vi "DestroyRequestEvents.vi"(8 "error in (no error)":errorcluster) -> (0 "error out":errorcluster)   [LabVIEW 2018, in "MyPlugins.lvlib"]
doc: "Closes the user events generated that describe which requests can be sent to the module."
uses:
  MyPlugins.lvlib
  PluginsShared/clRequestEvents.ctl
  PluginsShared/clEventType.ctl
  PluginsShared/PluginsShared.lvlib
panel:
  out "clRequestEvents":T1
  # "If you want to add other Request Events, open this typedef, copy an existing event and rename it to your Request name.\n\nNext create a typedef for the  data and put it into PublicAPI/Arguments/Requests\n\nNext, add an event handler loop event case in Main.vi to handle the new request event\n\nMost likely, each request will also require the creation of a new Queued Message Handler loop case in Main.VI"
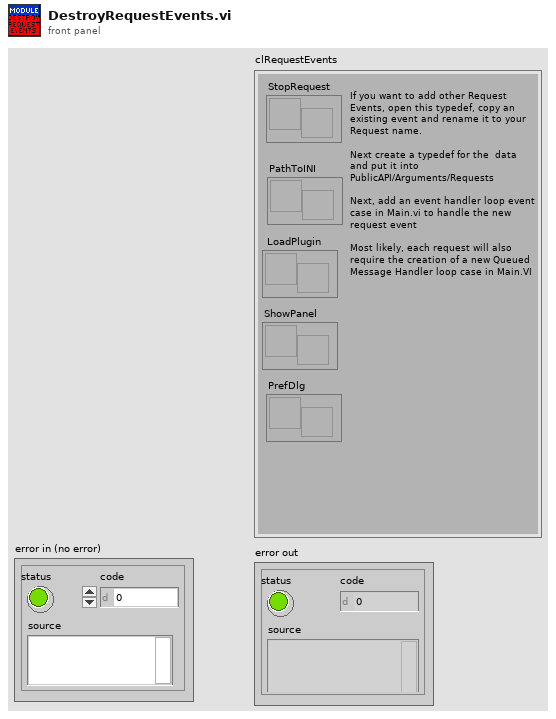
[diagram p1: front panel]
types:
  T1 = typedef "PluginsShared.lvlib/clRequestEvents.ctl" = cluster{"StopRequest":refnum<user-event>, "PathToINI":refnum<user-event>, " LoadPlugin":refnum<user-event>, "ShowPanel":refnum<user-event>, "PrefDlg":refnum<user-event>}
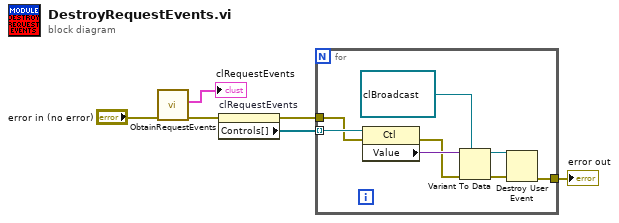
[diagram p0: block diagram]
diagram:
  n1 = call "ObtainRequestEvents.vi"("error in (no error)"="error in (no error)") -> ("error out"=w2:errorcluster, "clRequestEvents"=→"clRequestEvents":T1)  [unwired: 9 in]
  n2 = property on="clRequestEvents" class="Clust (strict)"(error in=w2) -> (error out=w1:errorcluster, "Controls[]"=w5:refnum<vi>[])  [unwired: 1 in, 1 out]
  n3 = for {
    tunnel: w5 -> [w14] mode=indexing
    tunnel: w1 -> [w8]
    tunnel: [w11] -> w6
    n4 = property class="Ctl"(reference=w14, error in=w8) -> (error out=w7:errorcluster, "Value"=w13:variant)  [unwired: 1 out]
    n5 = Variant To Data(error in=w7, type=refnum<user-event> refnum ("StopRequest"), Variant=w13) -> (data=w10:refnum<user-event>, error out=w12:errorcluster)
    n6 = Destroy User Event(user event=w10, error in=w12) -> (error out=w11:errorcluster)
  }
  "error out" <- w6
